vi "intersecBallVel.vi"(8 "error in (no error)":errorcluster, 10 "Game":refnum<class "Game.lvclass">, 11 "Utilities in":refnum<class "Utilities.lvclass">) -> (0 "error out":errorcluster, 1 "pos out":dbl[](array[numeric]), 2 "Game out":refnum<class "Game.lvclass">, 3 "Utilities out":refnum<class "Utilities.lvclass">)   [LabVIEW 2020, in "Utilities.lvclass"]
uses:
  Utilities.lvclass
  Game_class/Game.lvclass
  Game_class/Game.lvclass/Game.ctl
  Object_class/Object.lvclass/Object.ctl
  <vilib>/Analysis/_algsub.llb/Real Vector Norm.vi
  <vilib>/Analysis/baseanly.llb/Unit Vector (DBL).vi
  Game_class/Read BallRef.vi
  Game_class/Read FieldRef.vi
  Object_class/Read position(x,y).vi
  Ball_class/Ball.lvclass
  C:/Users/anton/Desktop/RoboIME/SSL_COMP/SSL_AI/Object_class/Object.lvclass
  Field_class/Field.lvclass
  <vilib>/Analysis/NI_AALBase.lvlib
  <vilib>/Analysis/NI_AALPro.lvlib
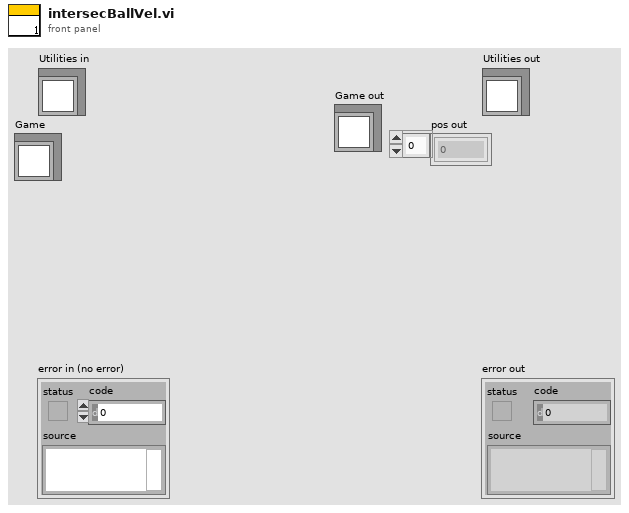
[diagram p1: front panel]
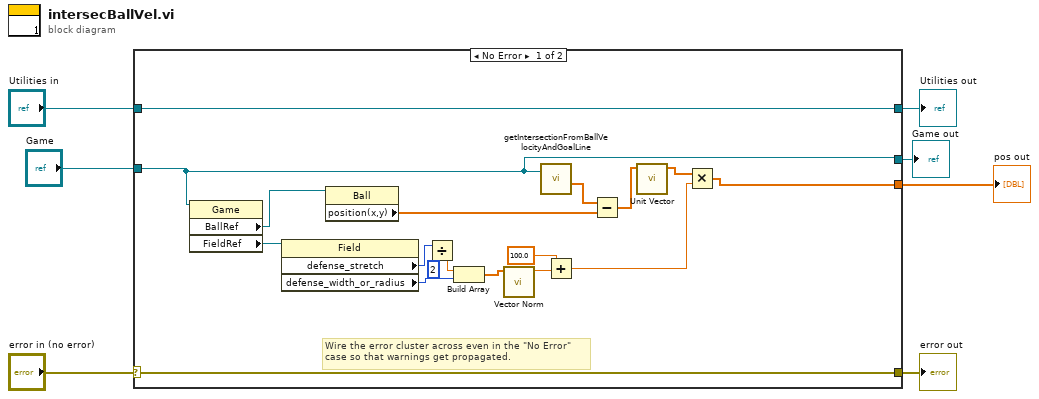
[diagram p0: block diagram]
diagram:
  n1 = case shown="No Error" "error in (no error)" {
    selector: "error in (no error)" -> [w24 w27]
    tunnel: [w24 w27] -> w6
    tunnel: [w25 w26] -> w4
    tunnel: "Utilities in" -> [w25 w26]
    tunnel: "Game" -> [w16 _]
    tunnel: [w17 _] -> w1
    tunnel: [w16 _] -> w2
    frame No Error {
      # "Wire the error cluster across even in the \"No Error\"\ncase so that warnings get propagated."
      n2 = property class="Game"(reference=w16) -> ("BallRef"=w14:refnum<class "Ball.lvclass">, "FieldRef"=w23:refnum<class "Field.lvclass">)  [unwired: 1 in, 2 out]
      n3 = property class="Field"(reference=w23) -> ("defense_stretch"=w10:i32, "defense_width_or_radius"=w22:i32)  [unwired: 1 in, 2 out]
      n4 = property class="Ball"(reference=w14) -> ("position(x,y)"=w12:dbl[])  [unwired: 1 in, 2 out]
      n5 = Divide(x=w10, y=2) -> (x/y=w8:dbl)
      n6 = Build Array(w8, w22) -> (w21:dbl[])
      n7 = call-poly <vilib>:"Vector Norm.vi"("Input Vector"=w21) -> ("norm"=w20:dbl)  [unwired: 9 in, 1 out]
      n8 = call "getIntersectionFromBallVelocityAndGoalLine.vi"("Game"=w16) -> ("Pos Out"=w13:dbl[])  [unwired: 8 in, 2 out]
      n9 = Add(x=100.0, y=w20) -> (x+y=w18:dbl)
      n10 = Subtract(x=w13, y=w12) -> (x-y=w11:dbl[])
      n11 = call-poly <vilib>:"Unit Vector.vi"("Input Vector"=w11) -> ("Unit Vector"=w15:dbl[])  [unwired: 8 in, 2 out]
      n12 = Multiply(x=w15, y=w18) -> (x*y=w17:dbl[])
    }
    frame Error {
    }
  }
  "error out" <- w6
  "Utilities out" <- w4
  "Game out" <- w2
  "pos out" <- w1
